vi "sub_stop-point_searching_currwpt.vi"(11 "waypoint in":cluster{"x":dbl, "y":dbl}[](array[cluster])) -> (3 "stop_point_buff":cluster{dbl, dbl}[](array[cluster]))   [LabVIEW 2019]
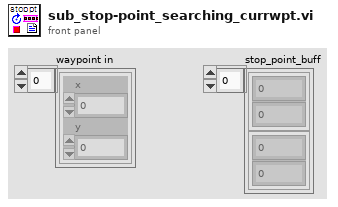
[diagram p1: front panel]
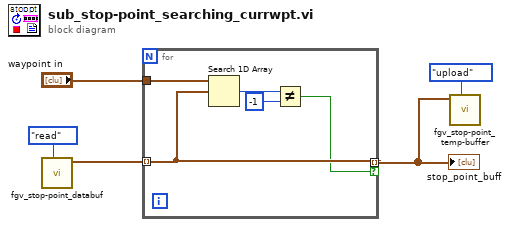
[diagram p0: block diagram]
diagram:
  n1 = call "fgv_stop-point_databuf.vi"("cmd"=enum16{"clear", "write", "read"}."read") -> ("all stop pts out"=w4:cluster{dbl, dbl}[])  [unwired: 9 in, 1 out]
  n2 = for {
    tunnel: w4 -> [w7] mode=indexing
    tunnel: "waypoint in" -> [w10]
    tunnel: [w7] -> w3 mode=indexing if=w6
    n3 = Search 1D Array(1D array=w10, element=w7) -> (index of element=w9:i32)  [unwired: 1 in]
    n4 = Not Equal?(x=w9, y=-1) -> (x != y?=w6:bool)
  }
  "stop_point_buff" <- w3
  n5 = call "fgv_stop-point_temp-buffer.vi"("cmd"=enum16{"init", "upload", "read", "del"}."upload", "stop pt array"=w3) -> ()  [unwired: 9 in, 1 out]
